vi "ProgressBar stopNotifier.vi"(8 "error in (no error)":errorcluster, 11 "ProgressBar in":refnum<class "ProgressBar.lvclass">) -> (0 "error out":errorcluster, 3 "ProgressBar out":refnum<class "ProgressBar.lvclass">)   [LabVIEW 2018, in "ProgressBar.lvclass"]
uses:
  ProgressBar.lvclass
  ProgressBar.lvclass/ProgressBar.ctl
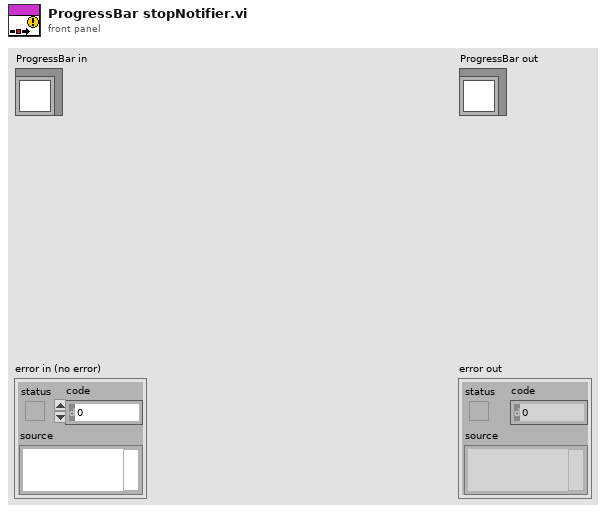
[diagram p1: front panel]
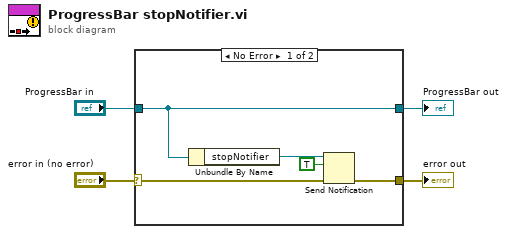
[diagram p0: block diagram]
diagram:
  n1 = case shown="No Error" "error in (no error)" {
    selector: "error in (no error)" -> [w6 w11]
    tunnel: [w5 w11] -> w1
    tunnel: [w9 w10] -> w2
    tunnel: "ProgressBar in" -> [w9 w10]
    frame No Error {
      n2 = Unbundle By Name(w9) -> ("stopNotifier"=w7:refnum<notifier>)
      n3 = Send Notification(notification=TRUE, notifier=w7, error in (no error)=w6) -> (error out=w5:errorcluster)  [unwired: 1 out]
    }
    frame Error {
    }
  }
  "error out" <- w1
  "ProgressBar out" <- w2
